vi "guardadoarchivocompleto.vi"(0 "nombre":string, 1 "lockin":dbl, 2 "multimetro":bool, 3 "CCD":dbl[][](array[numeric]), 5 "titulo grupo":string, 6 "voltaje":dbl, 7 "potenciometro":dbl, 8 "angulo":dbl, 9 "division":dbl, 10 "Enum":T1(ring), 11 "Orden":T2(array[ring])=[enum."espejos", enum."voltaje", enum."polarizador", enum."potenciometro "], 12 "polarizador":dbl, 13 "corriente":dbl, 14 "multim.":dbl) -> ()   [LabVIEW 2016]
doc: "En este subVI se realiza el guardado de la información de acuerdo con el dispositivo que se encuentre en penultimo lugar y si en ultimo lugar se encuentra la CCD. \n\nLas entradas son:\nLa cadena de nombre, en la que se especifica el nombre del archivo.\nLa cadena de nombre de los grupos que se van a realizar, en caso de que la cadena llegue vacía entoces no se forman ningún grupo."
uses:
  <vilib>/UPVI/lvhdf5/file.llb/LVH5F Operation.ctl
  <vilib>/Utility/miscctls.llb/LVRectTypeDef.ctl
  <vilib>/UPVI/lvhdf5/group.llb/H5G_obj_t.ctl
  <vilib>/UPVI/lvhdf5/dataset.llb/LVH5D Operation.ctl
  <vilib>/UPVI/lvhdf5/group.llb/OpenCreateGroup (String).vi
  <vilib>/UPVI/lvhdf5/utility.llb/Select HDF5 Dialog.vi
  <vilib>/UPVI/lvhdf5/utility.llb/Select HDF5 Dialog (Object Only).vi
  <vilib>/UPVI/lvhdf5/dataset.llb/Simple H5Dwrite (Variant).vi
  <vilib>/UPVI/lvhdf5/dataset.llb/Simple H5Dwrite.xnode
  <vilib>/UPVI/lvhdf5/library.llb/HDF5 Ref.ctl
  <vilib>/UPVI/lvhdf5/identifier.llb/Not an HDF5 Refnum Constant.vi
  <vilib>/Utility/error.llb/Error Cluster From Error Code.vi
  <vilib>/UPVI/lvhdf5/dataset.llb/OpenCreateReplace Dataset by Element Type.vi
  <vilib>/UPVI/lvhdf5/dataspace.llb/H5Sselect_hyperslab.vi
  <vilib>/UPVI/lvhdf5/dataset.llb/H5Dwrite (Variant).vi
  <vilib>/UPVI/lvhdf5/dataset.llb/H5Dget_space.vi
  <vilib>/UPVI/lvhdf5/attribute.llb/private/LVH5AwriteWDTAttrs.vi
  <vilib>/UPVI/lvhdf5/dataspace.llb/H5Sclose.vi
  <vilib>/UPVI/lvhdf5/dataset.llb/H5Dclose.vi
  <vilib>/UPVI/lvhdf5/utility.llb/Select HDF5 Dialog (File and Object).vi
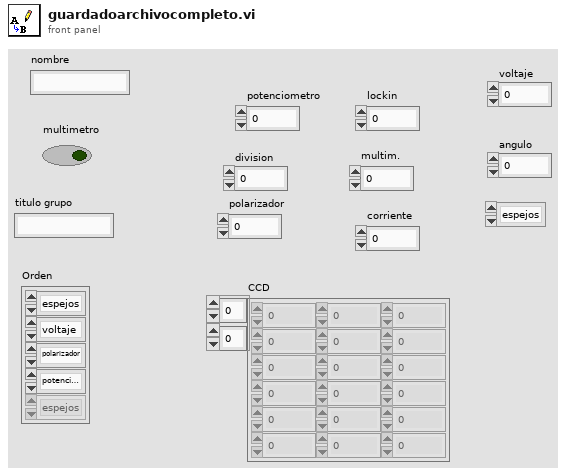
[diagram p1: front panel]
types:
  T1 = enum16{"espejos", "polarizador", "voltaje", "potenciometro ", "CCD", "lockin", "laser", "ninguno"}
  T2 = enum16{"espejos", "polarizador", "voltaje", "potenciometro ", "CCD", "lockin", "laser", "ninguno"}[]
  T3 = typedef "LVH5F Operation.ctl" = enum16{"open", "open or create", "create or replace", "create or replace (with confirmation)", "create", "open (read only)"}
  T4 = typedef "HDF5 Ref.ctl" = refnum<k1>
  T5 = typedef "LVRectTypeDef.ctl" = cluster{"Left":i16, "Top":i16, "Right":i16, "Bottom":i16}
  T6 = cluster{"Behavior":enum32{"Invalid", "Default", "Floating", "Floating/Auto-Hide", "Modal"}, "Position":T5, "Center":bool, "Title":string}
  T7 = typedef "LVH5D Operation.ctl" = enum16{"open", "replace", "create", "open or create", "create or replace", "create or replace with confirmation"}
  T8 = typedef "H5G_obj_t.ctl" = i32
  T9 = cluster{"Object Types (any)":T8[], "Object Pattern":string}
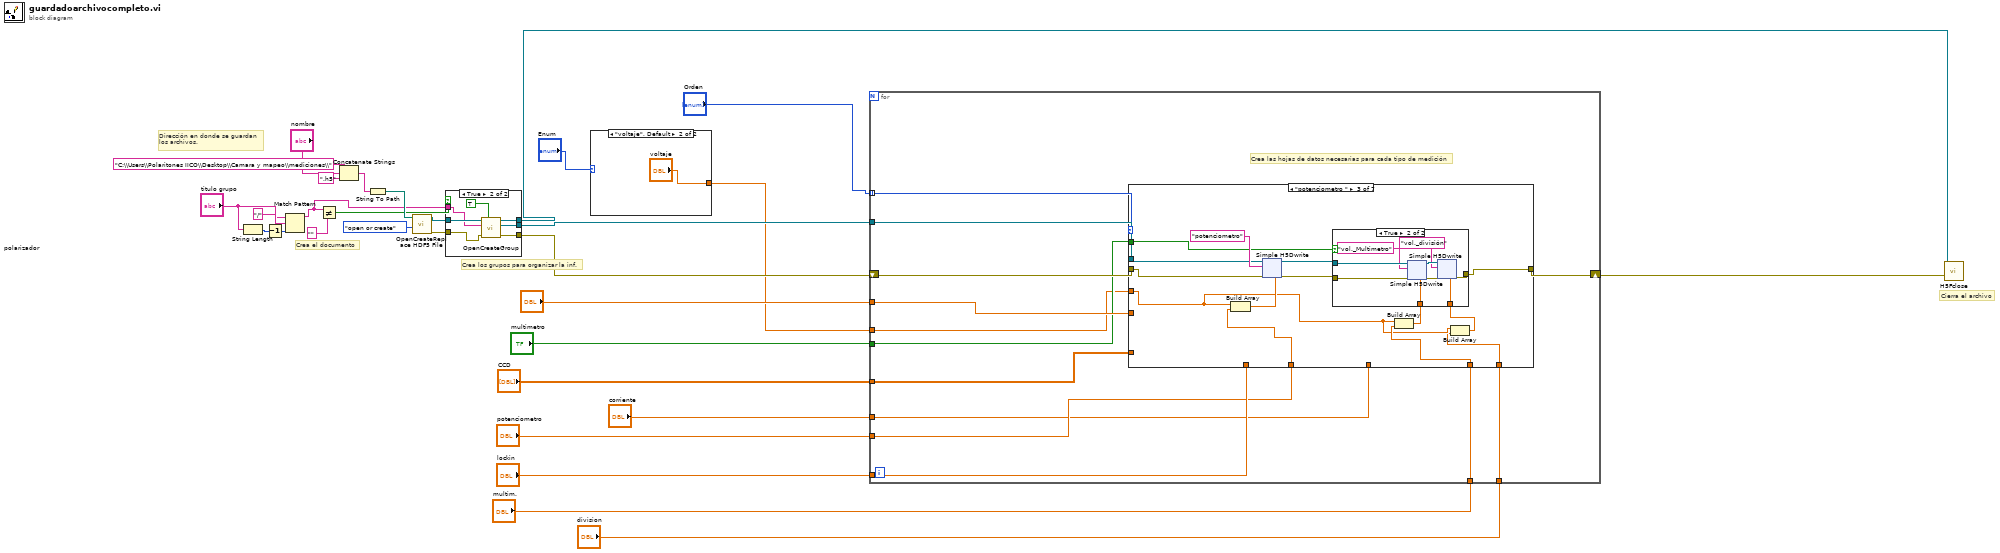
[diagram p0: block diagram]
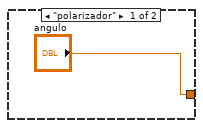
[diagram p2: hidden frame]
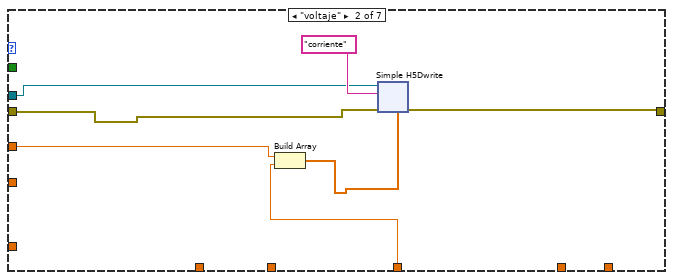
[diagram p4: hidden frame]
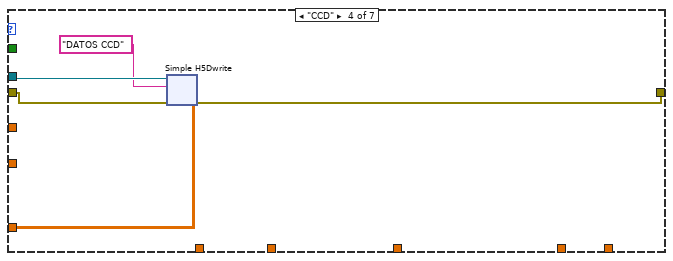
[diagram p6: hidden frame]
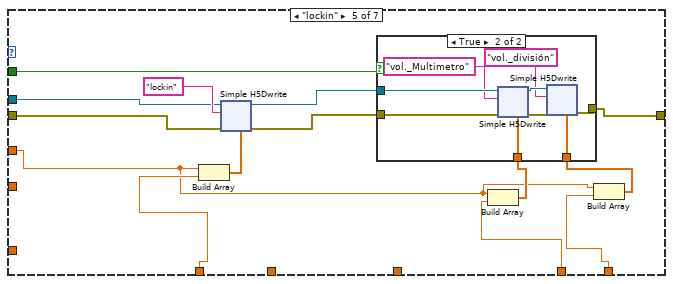
[diagram p7: hidden frame]
diagram:
  # "Dirección en donde se guardan \nlos archivos."
  # "Cierra el archivo"
  # "Crea los grupos para organizar la inf."
  # "Crea el documento"
  n1 = String Length(string="titulo grupo") -> (length=w12:i32)
  n2 = Decrement(x=w12) -> (x-1=w13:i32)
  n3 = Match Pattern(string="titulo grupo", regular expression="/", offset (0)=w13) -> (before substring=w8:string)  [unwired: 3 out]
  n4 = Not Equal?(x=w8, y="") -> (x != y?=w9:bool)
  n5 = Concatenate Strings("C:\\Users\\Polaritones IICO\\Desktop\\Camara y mapeo\\mediciones\\" ("string"), "nombre", ".h5" ("string")) -> (w24:string)
  n6 = String To Path(string=w24) -> (path=w23:path)
  n7 = call <vilib>:"OpenCreateReplace HDF5 File.vi"("function (open or create)"=LVH5F_Operation."open or create", "path"=w23) -> ("error out"=w28:errorcluster, "HDF5 Ref out"=w29:T4)  [unwired: 6 in]
  n8 = case shown="True" w9 {
    tunnel: w29 -> [w32 w39]
    tunnel: w28 -> [w31 w38]
    tunnel: [w31 w37] -> w22
    tunnel: [w32 w36] -> w20
    tunnel: [w32 w34] -> w19
    tunnel: w8 -> [_ w33]
    frame False {
    }
    frame True {
      n9 = call-poly <vilib>:"OpenCreateGroup.vi"("Create if not found (F)"=TRUE, "error in (no error)"=w38, "Group"=w33, "HDF5 Ref"=w39) -> ("error out"=w37:errorcluster, "HDF5 Group Ref"=w36:T4, "HDF5 Ref out"=w34:T4)  [unwired: 5 in]
    }
  }
  n10 = case shown="\"voltaje\", Default" "Enum" {
    tunnel: ["angulo" "voltaje"] -> w2
    frame "polarizador" {
    }
    frame "voltaje", Default {
    }
  }
  n11 = for {
    tunnel: "polarizador" -> [w53]
    tunnel: w20 -> [w52]
    tunnel: "Orden" -> [w51] mode=indexing
    tunnel: "lockin" -> [w49]
    tunnel: "potenciometro" -> [w48]
    tunnel: "corriente" -> [w47]
    tunnel: "multimetro" -> [w46]
    tunnel: "multim." -> [w45]
    tunnel: "CCD" -> [w44]
    shift-right: [w50] -> w18
    shift-left: w22 -> [w54]
    tunnel: "division" -> [w43]
    tunnel: w2 -> [w42]
    # "Crea las hojas de datos necesarias para cada tipo de medición"
    n12 = case shown="\"potenciometro \"" w51 {
      tunnel: w54 -> [w55 w61 w275 w898 w1113 w1732 w1733]
      tunnel: w53 -> [_ _ _ _ _ _ _]
      tunnel: w52 -> [_ w59 w276 w897 w1114 _ _]
      tunnel: [w55 w60 w273 w899 w1110 w1732 w1733] -> w50
      tunnel: w49 -> [_ _ _ _ w1108 _ _]
      tunnel: w48 -> [_ _ w271 _ _ _ _]
      tunnel: w47 -> [_ w57 _ _ _ _ _]
      tunnel: w46 -> [_ _ w272 _ w1109 _ _]
      tunnel: w45 -> [_ _ w269 _ w1106 _ _]
      tunnel: w44 -> [_ _ _ w895 _ _ _]
      tunnel: w43 -> [_ _ w266 _ w1104 _ _]
      tunnel: w42 -> [_ w58 w267 _ w1103 _ _]
      frame "espejos", Default {
      }
      frame "voltaje" {
        n13 = Build Array(w58, w57) -> (w56:dbl[])
        n14 = xnode "Simple H5Dwrite"("Dataset Path"="corriente", "error in (no error)"=w61, "HDF5 Path or Ref"=w59, "Data"=w56) -> ("error out"=w60:errorcluster)  [unwired: 4 in, 2 out]
      }
      frame "potenciometro " {
        n15 = Build Array(w267, w271) -> (w270:dbl[])
        n16 = xnode "Simple H5Dwrite"("Dataset Path"="potenciometro", "error in (no error)"=w275, "HDF5 Path or Ref"=w276, "Data"=w270) -> ("HDF5 Ref out"=w277:T4, "error out"=w274:errorcluster)  [unwired: 4 in, 1 out]
        n17 = Build Array(w267, w269) -> (w268:dbl[])
        n18 = Build Array(w267, w266) -> (w265:dbl[])
        n19 = case shown="True" w272 {
          tunnel: w274 -> [w481 w490]
          tunnel: w277 -> [_ w489]
          tunnel: [w481 w485] -> w273
          tunnel: w268 -> [_ w483]
          tunnel: w265 -> [_ w482]
          frame False {
          }
          frame True {
            n20 = xnode "Simple H5Dwrite"("Dataset Path"="vol._Multimetro", "error in (no error)"=w490, "HDF5 Path or Ref"=w489, "Data"=w483) -> ("HDF5 Ref out"=w486:T4, "error out"=w487:errorcluster)  [unwired: 4 in, 1 out]
            n21 = xnode "Simple H5Dwrite"("Dataset Path"="vol._división", "error in (no error)"=w487, "HDF5 Path or Ref"=w486, "Data"=w482) -> ("error out"=w485:errorcluster)  [unwired: 4 in, 2 out]
          }
        }
      }
      frame "CCD" {
        n22 = xnode "Simple H5Dwrite"("Dataset Path"="DATOS CCD", "error in (no error)"=w898, "HDF5 Path or Ref"=w897, "Data"=w895) -> ("error out"=w899:errorcluster)  [unwired: 4 in, 2 out]
      }
      frame "lockin" {
        n23 = Build Array(w1103, w1108) -> (w1107:dbl[])
        n24 = xnode "Simple H5Dwrite"("Dataset Path"="lockin", "error in (no error)"=w1113, "HDF5 Path or Ref"=w1114, "Data"=w1107) -> ("HDF5 Ref out"=w1112:T4, "error out"=w1111:errorcluster)  [unwired: 4 in, 1 out]
        n25 = Build Array(w1103, w1106) -> (w1105:dbl[])
        n26 = Build Array(w1103, w1104) -> (w1102:dbl[])
        n27 = case shown="True" w1109 {
          tunnel: w1111 -> [w1116 w1125]
          tunnel: w1112 -> [_ w1124]
          tunnel: [w1116 w1120] -> w1110
          tunnel: w1105 -> [_ w1118]
          tunnel: w1102 -> [_ w1117]
          frame False {
          }
          frame True {
            n28 = xnode "Simple H5Dwrite"("Dataset Path"="vol._Multimetro", "error in (no error)"=w1125, "HDF5 Path or Ref"=w1124, "Data"=w1118) -> ("HDF5 Ref out"=w1121:T4, "error out"=w1122:errorcluster)  [unwired: 4 in, 1 out]
            n29 = xnode "Simple H5Dwrite"("Dataset Path"="vol._división", "error in (no error)"=w1122, "HDF5 Path or Ref"=w1121, "Data"=w1117) -> ("error out"=w1120:errorcluster)  [unwired: 4 in, 2 out]
          }
        }
      }
      frame "laser" {
      }
      frame "ninguno" {
      }
    }
  }
  n30 = call <vilib>:"H5Fclose.vi"("error in (no error)"=w18, "HDF5 Ref"=w19) -> ()  [unwired: 7 in, 1 out]
